vi "CFG Load Tree.vi"(0 "Tree":refnum<vi>, 1 "Parameters In":T1[](array[typedef]), 11 "error in (no error)":errorcluster) -> (15 "error Out":errorcluster)   [LabVIEW 2017]
uses:
  Type Defs/CFG Key Cluster.ctl
  Type Defs/CFG Tag Type Enum.ctl
panel:
  in  "Tree":string(tree)
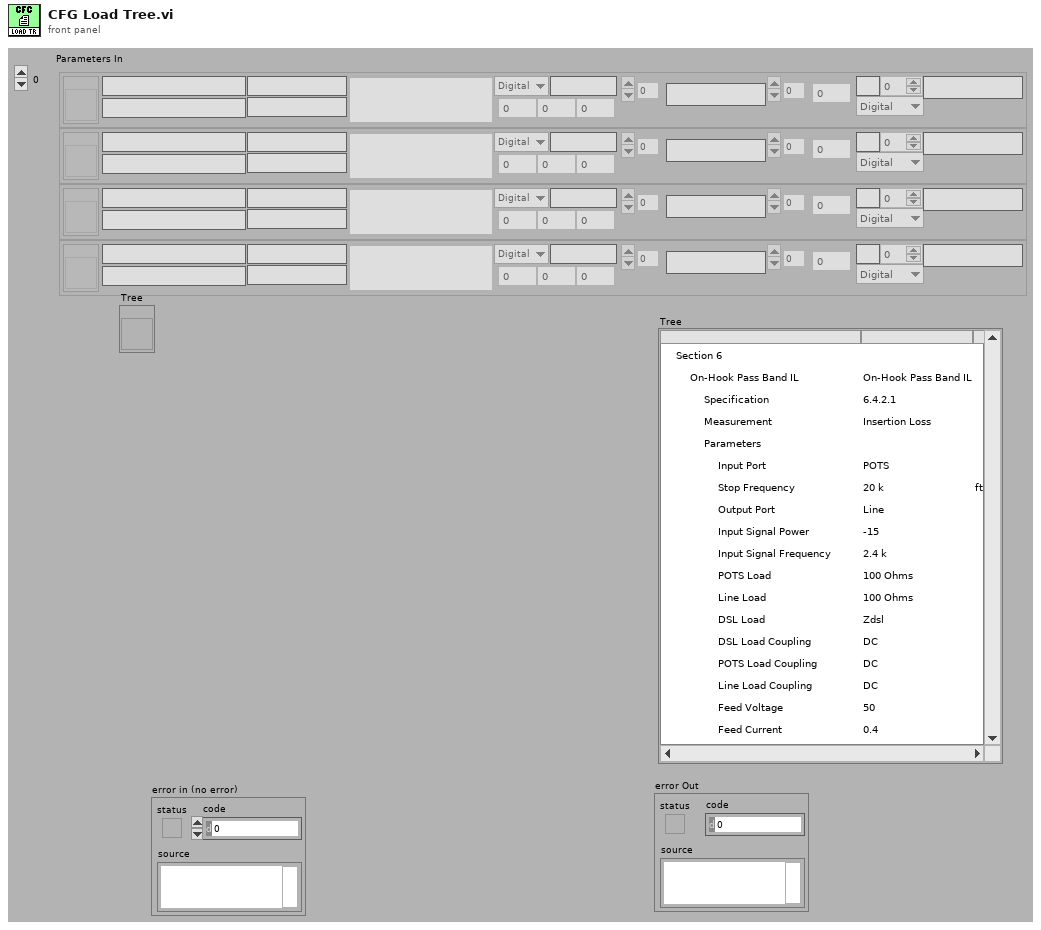
[diagram p1: front panel]
types:
  T1 = typedef "CFG Key Cluster.ctl" = cluster{"Strings []":string[], "Disabled Items []":i32[], "Value":variant, "Format String":string, "Tag":string, "Type":T2, "Section":string, " Ctl Ref":refnum<vi>, "Data Range":cluster{"Minimum":dbl, "Maximum":dbl, "Increment":dbl}, "Unit":string, "Special Instructions":string, "Delimiter(s)":string, "Dimensions":i32, "Element Type":T2, "Array Value String":string}
  T2 = typedef "CFG Tag Type Enum.ctl" = enum16{"Digital", "Slide", "Enum", "Boolean", "String", "Path", "Array", "VISAResourceName", "DAQmxName", "Cluster"}
  T3 = cluster{"Left Cell String":string, "Child Text":string[], "Child Tag":string, "Item Indent":i32, "Child Only?":bool, "Glyph Index":i32}
  T4 = cluster{"Left Cell String":string, "Child Text":string[], "Child Tag":string, "Item Indent":i32, "Child Only?":bool, "Glyph Index":i32}[]
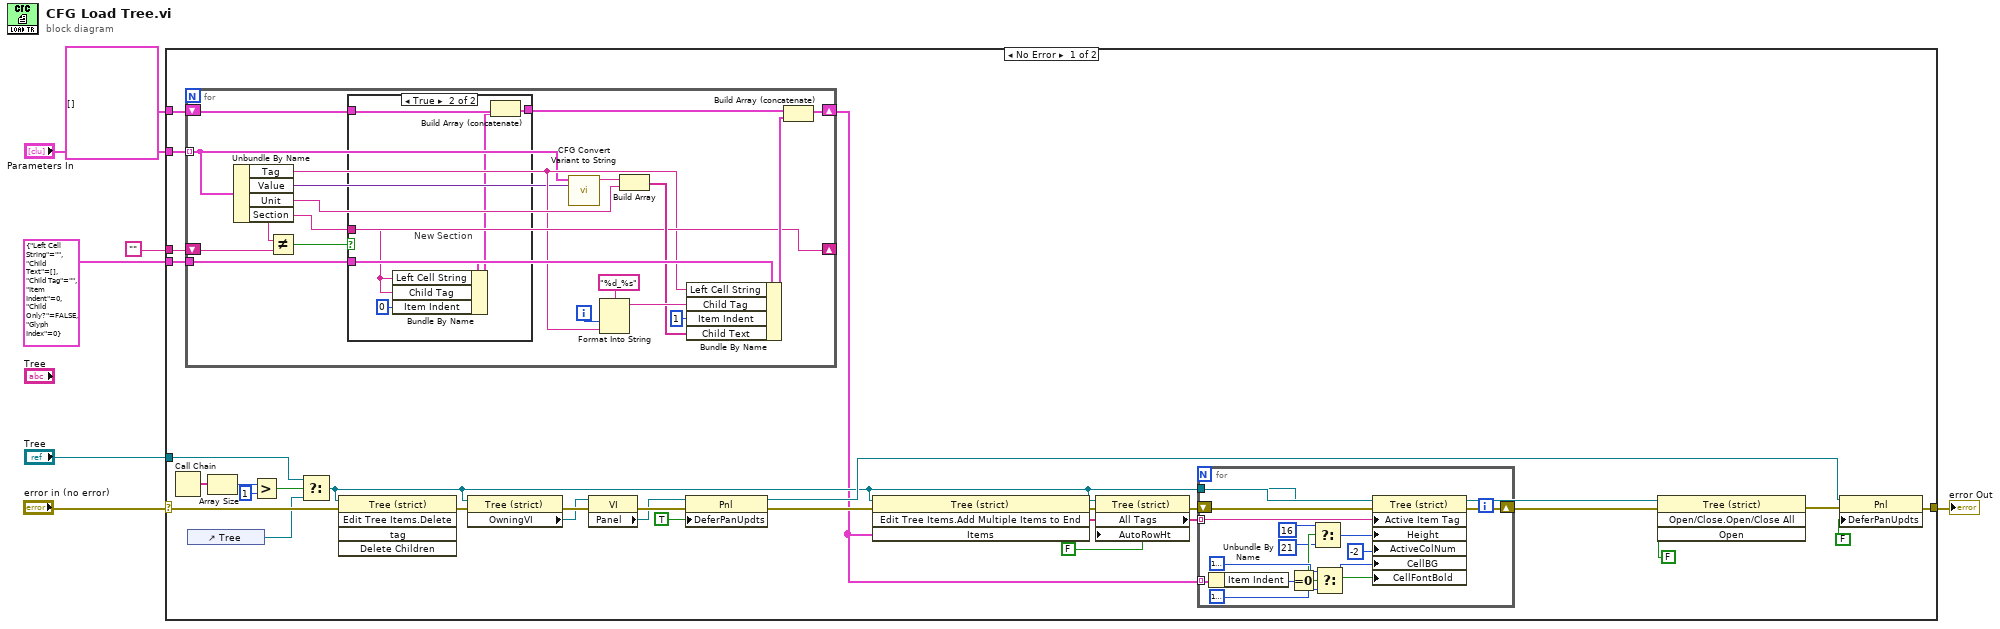
[diagram p0: block diagram]
diagram:
  n1 = case shown="No Error" "error in (no error)" {
    selector: "error in (no error)" -> [w34 w77]
    tunnel: [w21 w77] -> w2
    tunnel: "Parameters In" -> [w37 _]
    tunnel: T4 [] ("Items") -> [w36 _]
    tunnel: T3 {"Left Cell String"="", "Child Text"=[], "Child Tag"="", "Item Indent"=0, "Child Only?"=FALSE, "Glyph Index"=0} ("Item") -> [w35 _]
    tunnel: "Tree" -> [w29 _]
    tunnel: "" -> [w18 _]
    frame No Error {
      n2 = Call Chain() -> (call chain=w33:string[])
      n3 = for {
        tunnel: w37 -> [w57] mode=indexing
        shift-right: [w68] -> w8
        shift-left: w36 -> [w55]
        tunnel: w35 -> [w69]
        shift-right: [w60] -> _
        shift-left: w18 -> [w62]
        i -> [w53]
        n4 = Unbundle By Name(w57) -> ("Tag"=w59:string, "Value"=w58:variant, "Unit"=w67:string, "Section"=w60:string)
        n5 = Not Equal?(x=w60, y=w62) -> (x != y?=w61:bool)
        n6 = case shown="True" w61 {
          tunnel: w69 -> [_ w76]
          tunnel: w60 -> [_ w74]
          tunnel: w55 -> [w70 w73]
          tunnel: [w70 w72] -> w54
          frame False {
          }
          frame True {
            # "New Section"
            n7 = Bundle By Name(cluster=w76, "Left Cell String"=w74, "Child Tag"=w74, "Item Indent"=0) -> (w71:T3)
            n8 = Build Array (concatenate)(w73, w71) -> (w72:T4)
          }
        }
        n9 = call "CFG Convert Variant to String.vi"("Key Cluster"=w57, "Value (Variant)"=w58) -> ("Value (Str)"=w56:string)  [unwired: 1 in, 12 out]
        n10 = Format Into String(format string="%d_%s", w53, w59) -> (resulting string=w65:string)  [unwired: 2 in, 1 out]
        n11 = Build Array(w56, w67) -> (w64:string[])
        n12 = Bundle By Name(cluster=w69, "Left Cell String"=w59, "Child Tag"=w65, "Item Indent"=1, "Child Text"=w64) -> (w66:T3)
        n13 = Build Array (concatenate)(w54, w66) -> (w68:T4)
      }
      n14 = control-ref of="Tree"() -> (w28:refnum<vi>)
      n15 = Array Size(array=w33) -> (size(s)=w32:i32)
      n16 = Greater?(x=w32, y=1) -> (0:w30:bool)
      n17 = Select(t=w29, s=w30, f=w28) -> (s? t:f=w9:refnum<vi>)
      n18 = invoke on="Invoke Node" class="Tree (strict)" method="Edit Tree Items.Delete"(reference=w9, error in=w34) -> (error out=w23:errorcluster)  [unwired: 3 in, 4 out]
      n19 = property class="Tree (strict)"(reference=w9, error in=w23) -> (error out=w17:errorcluster, "OwningVI"=w15:refnum<vi>)  [unwired: 1 out]
      n20 = property class="VI"(reference=w15, error in=w17) -> (error out=w16:errorcluster, "Panel"=w14:refnum<vi>)  [unwired: 1 out]
      n21 = property class="Pnl"(reference=w14, error in=w16, "DeferPanUpdts"=TRUE ("Defer Panel Updates")) -> (reference out=w11:refnum<vi>, error out=w22:errorcluster)
      n22 = invoke on="Invoke Node" class="Tree (strict)" method="Edit Tree Items.Add Multiple Items to End"(reference=w9, error in=w22, "Items"=w8) -> (error out=w27:errorcluster, "Edit Tree Items:Add Multiple Items to End"=w25:string[])  [unwired: 1 in, 2 out]
      n23 = property class="Tree (strict)" props=["All Tags", "AutoRowHt"](reference=w9, error in=w27, "AutoRowHt"=FALSE ("Autosizing Row Height")) -> (error out=w26:errorcluster)  [unwired: 2 out]
      n24 = for {
        tunnel: w9 -> [w49]
        tunnel: w25 -> [w48] mode=indexing
        shift-right: [w50] -> w13
        shift-left: w26 -> [w51]
        tunnel: w8 -> [w44] mode=indexing
        n25 = Unbundle By Name(w44) -> ("Item Indent"=w43:i32)
        n26 = Equal To 0?(x=w43) -> (x = 0?=w40:bool)
        n27 = Select(t=16 ("Active Cell:Cell Size:Height"), s=w40, f=21 ("Active Cell:Cell Size:Height")) -> (s? t:f=w39:i32)
        n28 = Select(t=u32 16777226, s=w40, f=u32 16777238) -> (s? t:f=w42:u32)
        n29 = property class="Tree (strict)"(reference=w49, error in=w51, "Active Item Tag"=w48, "Height"=w39, "ActiveColNum"=-2 ("Active Cell:Active Column Number"), "CellBG"=w42, "CellFontBold"=w40) -> (error out=w50:errorcluster)  [unwired: 1 out]
      }
      n30 = invoke on="Invoke Node" class="Tree (strict)" method="Open/Close.Open/Close All"(reference=w9, error in=w13, "Open"=FALSE ("Open?")) -> (error out=w10:errorcluster)  [unwired: 1 in, 3 out]
      n31 = property class="Pnl"(reference=w11, error in=w10, "DeferPanUpdts"=FALSE ("Defer Panel Updates")) -> (error out=w21:errorcluster)  [unwired: 1 out]
    }
    frame Error {
    }
  }
  "error Out" <- w2
